vi "Create.vi"(8 "error in (no error)":errorcluster) -> (0 "error out":errorcluster, 3 "GA-Retract-Cmd out":refnum<class "GA-Retract-Cmd.lvclass">)   [LabVIEW 2013, in "GA-Retract-Cmd.lvclass"]
uses:
  GA-Retract-Cmd.lvclass
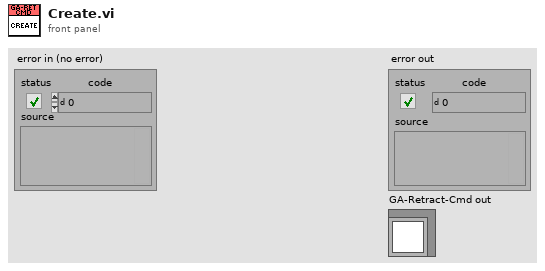
[diagram p1: front panel]
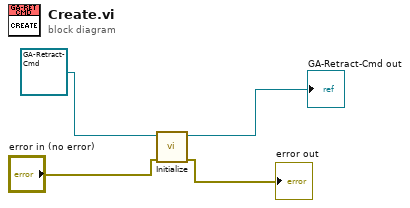
[diagram p0: block diagram]
diagram:
  n1 = call-dynamic "Initialize.vi"("error in (no error)"="error in (no error)", "GA-Retract-Cmd in"=refnum<class "GA-Retract-Cmd.lvclass"> refnum ("GA-Retract-Cmd.lvclass")) -> ("error out"=→"error out":errorcluster, "GA-Retract-Cmd out"=→"GA-Retract-Cmd out":refnum<class "GA-Retract-Cmd.lvclass">)  [unwired: 8 in]
